vi "Index Array Elements (2D) Example 01.vi"() -> ()   [LabVIEW 2020]
uses:
  <userlib>/_OpenG.lib/array/array.llb/Index 2D Array Elements (U32)__ogtk.vi
panel:
  in  "indices (1)":i32[](array[numeric])=[0, 2, 3]
  out "elements":u32[](array[colorbox])
  in  "indices (0)":i32[](array[numeric])=[0, 1, 2]
  in  "array":u32[][](array[colorbox])=[[16716306, 1250047, 65309, 16777215], [0, 5898232, 946944, 16716521], [12961221, 16775680, 10556159, 16758850]]
  # "<== These are the indices of elements from array, that you want to obtain in the elements array.  indices (0) are the rows and indices (1) are the columns."
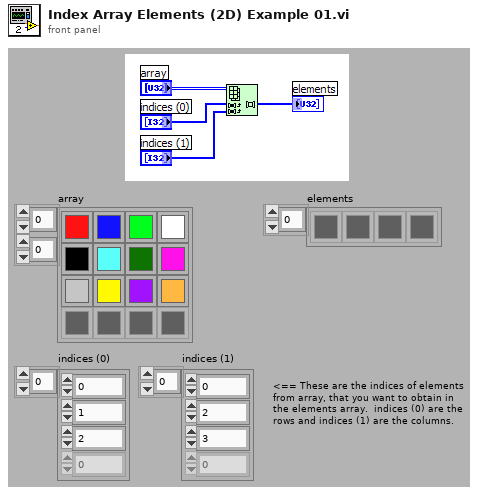
[diagram p1: front panel]
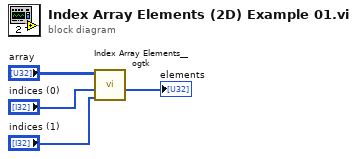
[diagram p0: block diagram]
diagram:
  n1 = call-poly <userlib>:"Index Array Elements__ogtk.vi"("indices 1"="indices (1)", "indices 0"="indices (0)", "array"="array") -> ("elements"=→"elements":u32[])  [unwired: 8 in]
